vi "Generic Arcade.vi"(5 "Lock":string, 7 "Force? (F)":bool, 8 "error in (no error)":errorcluster, 9 "Y Axis":dbl, 10 "X Axis":dbl, 11 "Queue in":refnum<queue>) -> (0 "error out":errorcluster, 3 "queue out":refnum<queue>)   [LabVIEW 2016, in "Drive System.lvlib"]
uses:
  Drive System.lvlib
  DriveCmd.ctl
  DriveCmdList.ctl
  Varient Cmd Types/Drive Arcade.ctl
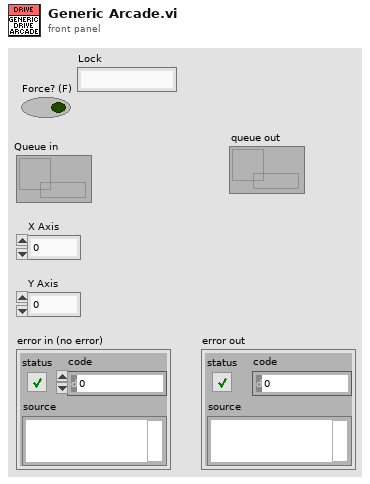
[diagram p1: front panel]
types:
  T1 = typedef "Drive System.lvlib/Drive Arcade.ctl" = cluster{"X Axis":dbl, "Y Axis":dbl}
  T2 = typedef "Drive System.lvlib/DriveCmd.ctl" = cluster{"cmd":T3, "data":variant, "Force? (F)":bool, "Lock":string}
  T3 = typedef "Drive System.lvlib/DriveCmdList.ctl" = enum16{"Idle", "Cleanup", "Drive For Time", "Drive Tank", "Drive Arcade", "Unlock", "Lock"}
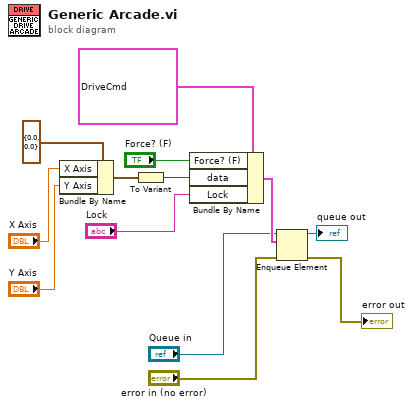
[diagram p0: block diagram]
diagram:
  n1 = Bundle By Name(cluster=T1 {"X Axis"=0.0, "Y Axis"=0.0} ("Cluster"), "X Axis"="X Axis", "Y Axis"="Y Axis") -> (w9:T1)
  n2 = To Variant(anything=w9) -> (Variant=w10:variant)
  n3 = Bundle By Name(cluster=T2 {"cmd"=enum."Drive Arcade", "data"=variant, "Force? (F)"=FALSE, "Lock"=""} ("element"), "Force? (F)"="Force? (F)", "data"=w10, "Lock"="Lock") -> (w13:T2)
  n4 = Enqueue Element(queue="Queue in", element=w13, error in (no error)="error in (no error)") -> (queue out=→"queue out":refnum<queue>, error out=→"error out":errorcluster)  [unwired: 1 in, 1 out]
